vi "Measurement-CC.vi"(2 "Ctl Refnum 2":refnum<vi>, 6 "开始频率":dbl[](array[numeric])=[20.0, 5000000.0, 100.0], 7 "Scanning Mode":u16(ring)=1 items=["Linear", "Log"], 8 "error in (no error)":errorcluster, 9 "Ctl Refnum":refnum<vi>, 10 "BSFR":refnum<file>, 11 "电阻地址":refnum<visa-resource-name>) -> (3 "Cluster":T1)   [LabVIEW 2017]
panel:
  out "电抗":dbl
  out "电阻":dbl
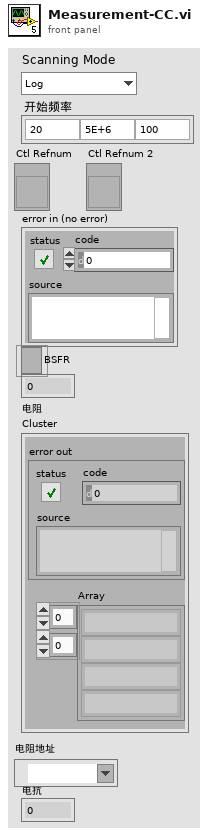
[diagram p1: front panel]
types:
  T1 = cluster{"Array":string[][], "error out":errorcluster}
  T2 = cluster{"Array 2":string[][], "error out":errorcluster}
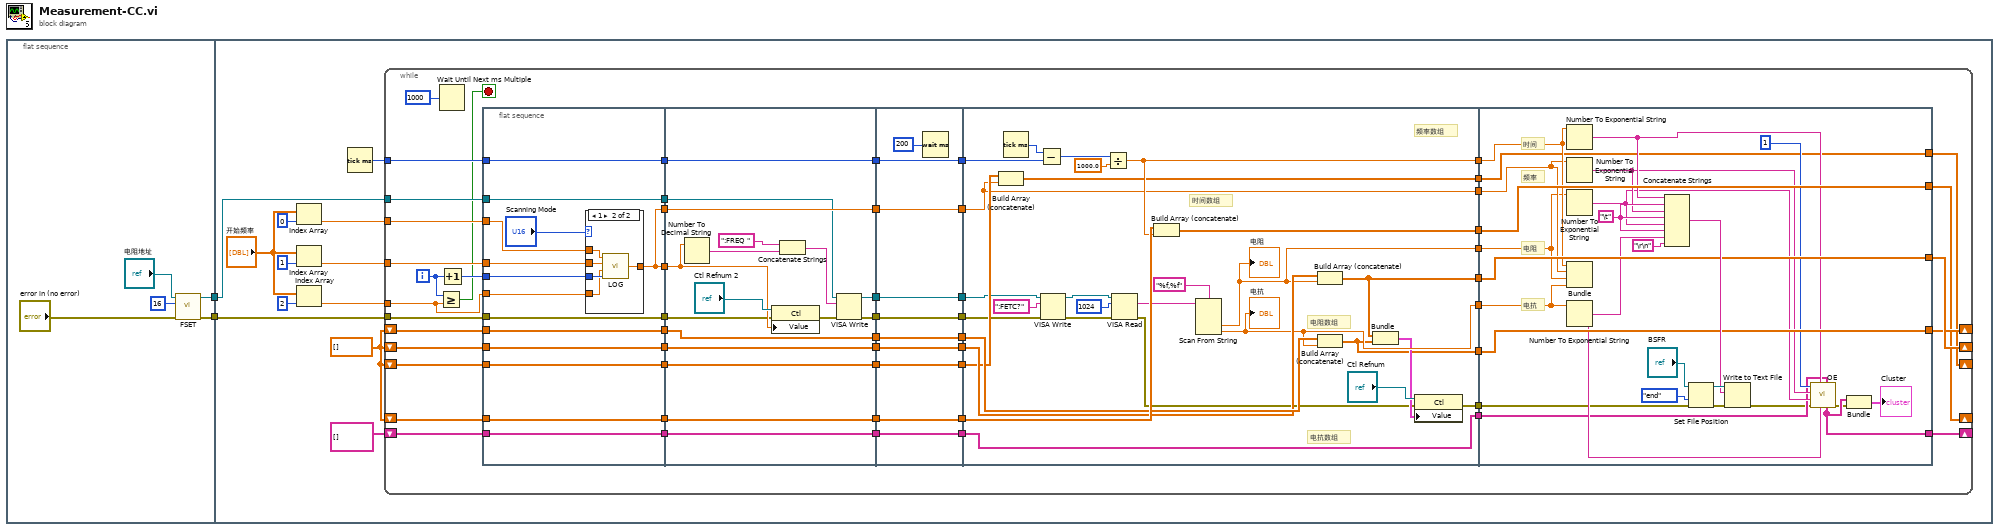
[diagram p0: block diagram]
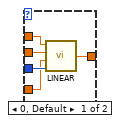
[diagram p2: hidden frame]
diagram:
  n1 = flat-sequence {
    tunnel: [w6] -> w2
    tunnel: [w5] -> w1
    tunnel: w2 -> [w18]
    tunnel: w1 -> [w17]
    frame #0 {
      n2 = call "FSET.vi"("error in (no error)"="error in (no error)", "Function (0: Cp-D)"=16, "VISA resource name"="电阻地址") -> ("error out"=w5:errorcluster, "VISA resource name out"=w6:refnum<visa-resource-name>)  [unwired: 7 in]
    }
    frame #1 {
      w15 = dbl[] []
      n3 = Index Array(array="开始频率", index=0 ("索引")) -> (element=w10:dbl)
      n4 = Index Array(array="开始频率", index=1 ("索引")) -> (element=w9:dbl)
      n5 = Index Array(array="开始频率", index=2 ("索引")) -> (element=w8:dbl)
      n6 = Tick Count (ms)() -> (millisecond timer value=w19:u32)
      n7 = while {
        tunnel: w19 -> [w77]
        shift-right: [w71] -> _
        shift-left: w15 -> [w76]
        shift-right: [w72] -> _
        shift-left: w15 -> [w75]
        shift-right: [w73] -> _
        shift-left: w15 -> [w74]
        tunnel: w18 -> [w63]
        tunnel: w17 -> [w62]
        shift-right: [w60] -> _
        shift-left: string[][] [] -> [w58]
        shift-right: [w57] -> _
        shift-left: w15 -> [w55]
        tunnel: w10 -> [w52]
        tunnel: w9 -> [w51]
        tunnel: w8 -> [w49]
        i -> [w50]
        stop <- w48 stop-if-true
        n8 = Greater Or Equal?(x=w50, y=w49) -> (x >= y?=w48:bool)
        n9 = Wait Until Next ms Multiple(millisecond multiple=u32 1000 ("毫秒倍数")) -> ()  [unwired: 1 out]
        n10 = Increment(x=w50) -> (x+1=w53:i32)
        n11 = flat-sequence {
          tunnel: w55 -> [w84]
          tunnel: w58 -> [w85]
          tunnel: w62 -> [w86]
          tunnel: w63 -> [w87]
          tunnel: w74 -> [w88]
          tunnel: w75 -> [w89]
          tunnel: w76 -> [w90]
          tunnel: w77 -> [w91]
          tunnel: [w91] -> w39
          tunnel: [w90] -> w37
          tunnel: [w89] -> w35
          tunnel: [w88] -> w33
          tunnel: [w87] -> w31
          tunnel: [w86] -> w29
          tunnel: [w85] -> w27
          tunnel: [w84] -> w25
          tunnel: w53 -> [w82]
          tunnel: w52 -> [w81]
          tunnel: w51 -> [w80]
          tunnel: w49 -> [w79]
          tunnel: [w78] -> w23
          tunnel: [w78] -> w20
          tunnel: w39 -> [w118]
          tunnel: [w118] -> w38
          tunnel: w37 -> [w117]
          tunnel: [w117] -> w36
          tunnel: w35 -> [w116]
          tunnel: [w116] -> w34
          tunnel: w33 -> [w115]
          tunnel: [w115] -> w32
          tunnel: w31 -> [w108]
          tunnel: [w107] -> w30
          tunnel: w29 -> [w103]
          tunnel: [w106] -> w28
          tunnel: w27 -> [w114]
          tunnel: [w114] -> w26
          tunnel: w25 -> [w113]
          tunnel: [w113] -> w24
          tunnel: w23 -> [w104]
          tunnel: [w110] -> w21
          tunnel: w20 -> [w110]
          tunnel: w38 -> [w128]
          tunnel: [w128] -> w47
          tunnel: w36 -> [w127]
          tunnel: [w127] -> w46
          tunnel: w34 -> [w126]
          tunnel: [w126] -> w45
          tunnel: w32 -> [w125]
          tunnel: [w125] -> w44
          tunnel: w30 -> [w124]
          tunnel: [w124] -> w41
          tunnel: w28 -> [w123]
          tunnel: [w123] -> w40
          tunnel: w26 -> [w122]
          tunnel: [w122] -> w43
          tunnel: w24 -> [w121]
          tunnel: [w121] -> w42
          tunnel: [w119] -> w22
          tunnel: w21 -> [w119]
          tunnel: [w129] -> w70
          tunnel: [w130] -> w69
          tunnel: [w150] -> w68
          tunnel: [w147] -> w67
          tunnel: [w146] -> w66
          tunnel: [w149] -> w65
          tunnel: [w131] -> w64
          tunnel: w47 -> [w156]
          tunnel: w46 -> [w153]
          tunnel: w45 -> [w152]
          tunnel: w44 -> [w151]
          tunnel: [w140] -> w59
          tunnel: w43 -> [w140]
          tunnel: [w139] -> w56
          tunnel: w42 -> [w138]
          tunnel: [w137] -> w54
          tunnel: w40 -> [w136]
          tunnel: w41 -> [w134]
          tunnel: w22 -> [w131]
          tunnel: [w179] -> w73
          tunnel: w70 -> [w179]
          tunnel: [w178] -> w72
          tunnel: w69 -> [w178]
          tunnel: [w177] -> w71
          tunnel: w68 -> [w177]
          tunnel: w67 -> [w171]
          tunnel: w66 -> [w170]
          tunnel: w65 -> [w173]
          tunnel: w64 -> [w172]
          tunnel: [w162] -> w60
          tunnel: w59 -> [w164]
          tunnel: [w158] -> w57
          tunnel: w56 -> [w158]
          tunnel: w54 -> [w161]
          frame #0 {
            n12 = case shown="1" "Scanning Mode" {
              tunnel: w82 -> [w96 w101]
              tunnel: w79 -> [w95 w100]
              tunnel: w81 -> [w94 w99]
              tunnel: w80 -> [w93 w98]
              tunnel: [w92 w97] -> w78
              frame 0, Default {
                n13 = call "LINEAR.vi"("I"=w96, "N"=w95, "END"=w93, "INITIAL"=w94) -> ("数值"=w92:dbl)
              }
              frame 1 {
                n14 = call "LOG.vi"("I"=w101, "N"=w100, "END"=w98, "INITIAL"=w99) -> ("数值"=w97:dbl)
              }
            }
          }
          frame #1 {
            n15 = Number To Decimal String(number=w104) -> (decimal integer string=w112:string)  [unwired: 1 in]
            n16 = property class="Ctl"(reference="Ctl Refnum 2", error in=w103, "Value"=w104) -> (error out=w102:errorcluster)  [unwired: 1 out]
            n17 = Concatenate Strings(":FREQ " ("字符串"), w112) -> (w109:string)
            n18 = VISA Write(VISA resource name=w108, write buffer=w109, error in (no error)=w102) -> (VISA resource name out=w107:refnum<visa-resource-name>, error out=w106:errorcluster)  [unwired: 1 out]
          }
          frame #2 {
            n19 = Wait (ms)(milliseconds to wait=u32 200 ("等待时间（毫秒）")) -> ()  [unwired: 1 out]
          }
          frame #3 {
            # "频率数组"
            # "电阻数组"
            # "电抗数组"
            # "时间数组"
            n20 = Build Array (concatenate)(w138, w131) -> (w139:dbl[])
            n21 = Tick Count (ms)() -> (millisecond timer value=w157:u32)
            n22 = Subtract(x=w157, y=w156) -> (x-y=w155:u32)
            n23 = VISA Write(VISA resource name=w134, write buffer=":FETC?", error in (no error)=w136) -> (VISA resource name out=w132:refnum<visa-resource-name>, error out=w133:errorcluster)  [unwired: 1 out]
            n24 = Divide(x=w155, y=1000.0) -> (x/y=w149:dbl)
            n25 = VISA Read(VISA resource name=w132, byte count=1024, error in (no error)=w133) -> (read buffer=w142:string, error out=w141:errorcluster)  [unwired: 2 out]
            n26 = Build Array (concatenate)(w153, w149) -> (w150:dbl[])
            n27 = Scan From String(format string="%f,%f" ("格式字符串"), input string=w142) -> (output 1=w147:dbl, output 2=w146:dbl)  [unwired: 4 in, 3 out]
            "电阻" <- w147
            "电抗" <- w146
            n28 = Build Array (concatenate)(w151, w147) -> (w129:dbl[])
            n29 = Build Array (concatenate)(w152, w146) -> (w130:dbl[])
            n30 = Bundle(w129, w130) -> (w144:cluster{dbl[], dbl[]})  [unwired: 1 in]
            n31 = property class="Ctl"(reference="Ctl Refnum", error in=w141, "Value"=w144) -> (error out=w137:errorcluster)  [unwired: 1 out]
          }
          frame #4 {
            w174 = "\t"
            # "频率"
            # "电抗"
            # "电阻"
            # "时间"
            n32 = Number To Exponential String(number=w173) -> (E-format string=w168:string)  [unwired: 3 out]
            n33 = Number To Exponential String(number=w172) -> (E-format string=w167:string)  [unwired: 3 out]
            n34 = Number To Exponential String(number=w171) -> (E-format string=w166:string)  [unwired: 3 out]
            n35 = Bundle(w173, "数值"=w172, "电阻"=w171, "电抗"=w170) -> ()  [unwired: 1 in, 1 out]
            n36 = Number To Exponential String(number=w170) -> (E-format string=w165:string)  [unwired: 1 in, 2 out]
            n37 = Concatenate Strings(w168, w174, w167, w174, w166, w174, w165, "\r\n") -> (w181:string)
            n38 = Set File Position(refnum="BSFR", from (0:start)=enum16{"start", "end", "current"}."end" ("自（0:起始）"), error in=w161) -> (refnum out=w183:refnum<file>, error out=w180:errorcluster)  [unwired: 1 out]
            n39 = Write to Text File(file (use dialog)=w183, text=w181, error in=w180) -> (error out=w159:errorcluster)  [unwired: 3 out]
            n40 = call "OE.vi"("Array"=w164, "String 4"=w165, "String"=w168, "error in (no error)"=w159, "String 3"=w166, "String 2"=w167, "Numeric"=1) -> ("error out"=w160:errorcluster, "Array 2"=w162:string[][])  [unwired: 2 in, 1 out]
            n41 = Bundle("Array 2"=w162, "error out"=w160) -> (→"Cluster":T2)  [unwired: 1 in]
          }
        }
      }
    }
  }
